vi "003 shift register led.vi"() -> ()   [LabVIEW 2019]
panel:
  in  "milliseconds to wait":u32(knob) max=1000 step=10 scale=0.0..1000.0
  out "Boolean":bool
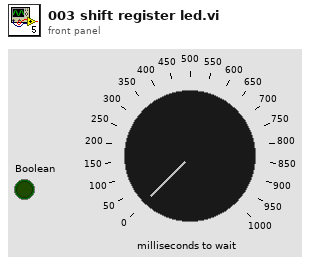
[diagram p1: front panel]
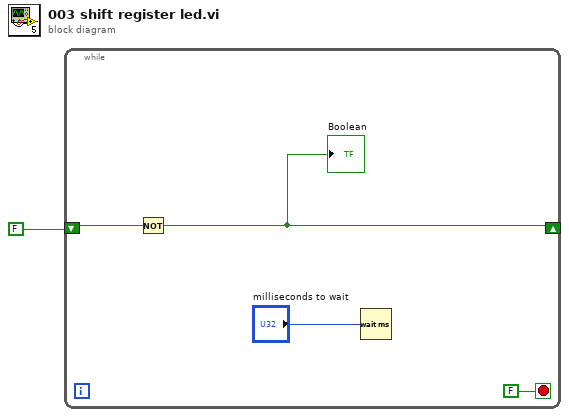
[diagram p0: block diagram]
diagram:
  n1 = while {
    shift-right: [w3] -> _
    shift-left: FALSE -> [w4]
    stop <- FALSE stop-if-true
    n2 = Not(x=w4) -> (.not. x?=w3:bool)
    "Boolean" <- w3
    n3 = Wait (ms)(milliseconds to wait="milliseconds to wait") -> ()  [unwired: 1 out]
  }
